vi "UpdatePortName.vi"(10 "ItemNames":string[](array[string]), 11 "Name":string) -> ()   [LabVIEW 2016]
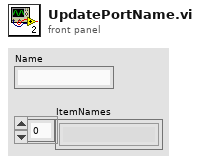
[diagram p1: front panel]
types:
  T1 = cluster{"Port Name":string, "Your Name":string}[]
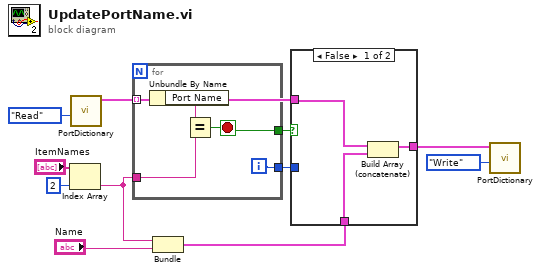
[diagram p0: block diagram]
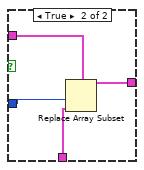
[diagram p2: hidden frame]
diagram:
  n1 = Index Array(array="ItemNames", index=2) -> (element=w4:string)
  n2 = call "PortDictionary.vi"("Tasks"=enum16{"Read", "Write"}."Read") -> ("Ports out"=w6:T1)  [unwired: 10 in]
  n3 = for {
    tunnel: w6 -> [w16] mode=indexing
    tunnel: w4 -> [w12]
    tunnel: [w15] -> w8
    tunnel: [w14] -> w7
    i -> [w14]
    stop <- w15 stop-if-true
    n4 = Unbundle By Name(w16) -> ("Port Name"=w13:string)
    n5 = Equal?(x=w13, y=w12) -> (x = y?=w15:bool)
  }
  n6 = Bundle(w4, "Name"="Name") -> (w3:cluster{string, "Name":string})  [unwired: 1 in]
  n7 = case shown="False" w8 {
    tunnel: w7 -> [_ w22]
    tunnel: w6 -> [w19 w23]
    tunnel: w3 -> [w18 w21]
    tunnel: [w17 w20] -> w1
    frame False {
      n8 = Build Array (concatenate)(w19, w18) -> (w17:cluster{"Port Name":string, "Name":string}[])
    }
    frame True {
      n9 = Replace Array Subset(array=w23, new element=w21, index=w22) -> (w20:T1)
    }
  }
  n10 = call "PortDictionary.vi"("Tasks"=enum16{"Read", "Write"}."Write", "Ports in"=w1) -> ()  [unwired: 9 in, 1 out]
